vi "Set Alternating BD Colours.vi"(8 "error in (no error)":errorcluster, 11 "VI Path":path) -> (0 "error out":errorcluster)   [LabVIEW 2020]
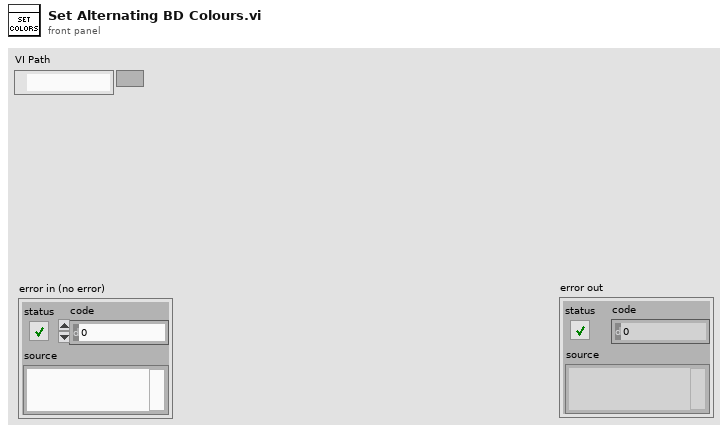
[diagram p1: front panel]
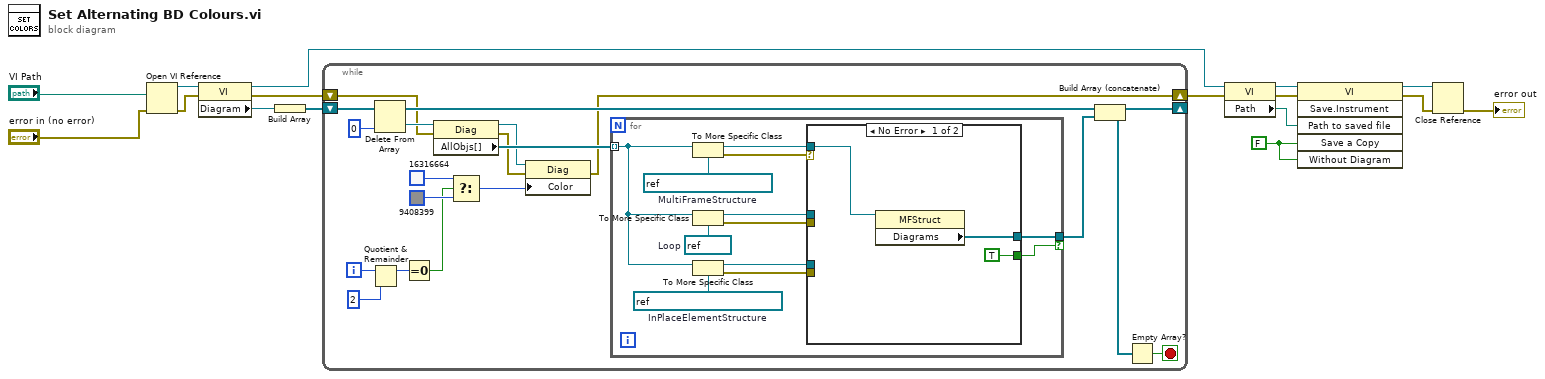
[diagram p0: block diagram]
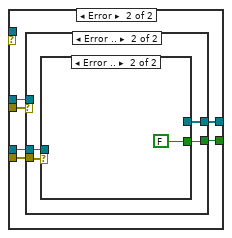
[diagram p2: hidden frame]
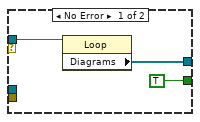
[diagram p3: hidden frame]
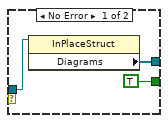
[diagram p4: hidden frame]
diagram:
  w5 = FALSE
  n1 = Open VI Reference(vi path="VI Path", error in (no error)="error in (no error)") -> (vi reference=w15:refnum<vi>, error out=w12:errorcluster)  [unwired: 4 in]
  n2 = property class="VI"(reference=w15, error in=w12) -> (reference out=w9:refnum<vi>, error out=w11:errorcluster, "Diagram"=w14:refnum<vi>)
  n3 = Build Array(w14) -> (w13:refnum<vi>[])
  n4 = while {
    shift-right: [w28] -> _
    shift-left: w13 -> [w35]
    shift-right: [w17] -> w10
    shift-left: w11 -> [w19]
    i -> [w27]
    stop <- w29 stop-if-true
    n5 = Quotient & Remainder(x=w27, y=2) -> (x-y*floor(x/y)=w23:i32)  [unwired: 1 out]
    n6 = Delete From Array(array=w35, index=0) -> (deleted portion=w33:refnum<vi>, array with subset deleted=w31:refnum<vi>[])  [unwired: 1 in]
    n7 = Equal To 0?(x=w23) -> (x = 0?=w22:bool)
    n8 = property class="Diag"(reference=w33, error in=w19) -> (reference out=w21:refnum<vi>, error out=w18:errorcluster, "AllObjs[]"=w32:refnum<vi>[])
    n9 = Select(t=u32 16316664, s=w22, f=u32 9408399) -> (s? t:f=w20:u32)
    n10 = property class="Diag"(reference=w21, error in=w18, "Color"=w20) -> (error out=w17:errorcluster)  [unwired: 1 out]
    n11 = for {
      tunnel: w32 -> [w44] mode=indexing
      tunnel: [w37] -> w30 if=w36
      w45 = refnum<vi> refnum  # InPlaceElementStructure
      w46 = refnum<vi> refnum  # Loop
      w47 = refnum<vi> refnum  # MultiFrameStructure
      n12 = To More Specific Class(target class=w47, reference=w44) -> (specific class reference=w42:refnum<vi>, error out=w43:errorcluster)  [unwired: 1 in]
      n13 = To More Specific Class(target class=w46, reference=w44) -> (specific class reference=w40:refnum<vi>, error out=w41:errorcluster)  [unwired: 1 in]
      n14 = To More Specific Class(target class=w45, reference=w44) -> (specific class reference=w38:refnum<vi>, error out=w39:errorcluster)  [unwired: 1 in]
      n15 = case shown="No Error" w43 {
        tunnel: w42 -> [w50 _]
        tunnel: w41 -> [_ w56]
        tunnel: w40 -> [_ w55]
        tunnel: w39 -> [_ w52]
        tunnel: w38 -> [_ w51]
        tunnel: [w49 w54] -> w37
        tunnel: [TRUE w53] -> w36
        frame No Error {
          n16 = property class="MFStruct"(reference=w50) -> ("Diagrams"=w49:refnum<vi>[])  [unwired: 1 in, 2 out]
        }
        frame Error {
          n17 = case shown="Error .." w56 {
            tunnel: w55 -> [w59 _]
            tunnel: [w58 w61] -> w54
            tunnel: [TRUE w60] -> w53
            tunnel: w52 -> [_ w63]
            tunnel: w51 -> [_ w62]
            frame No Error {
              n18 = property class="Loop"(reference=w59) -> ("Diagrams"=w58:refnum<vi>[])  [unwired: 1 in, 2 out]
            }
            frame Error {
              n19 = case shown="Error .." w63 {
                tunnel: w62 -> [w66 _]
                tunnel: [w65 _] -> w61
                tunnel: [TRUE FALSE] -> w60
                frame No Error {
                  n20 = property class="InPlaceStruct"(reference=w66) -> ("Diagrams"=w65:refnum<vi>[])  [unwired: 1 in, 2 out]
                }
                frame Error {
                }
              }
            }
          }
        }
      }
    }
    n21 = Build Array (concatenate)(w31, w30) -> (w28:refnum<vi>[])
    n22 = Empty Array?(array=w28) -> (empty?=w29:bool)
  }
  n23 = property class="VI"(reference=w9, error in=w10) -> (reference out=w7:refnum<vi>, error out=w8:errorcluster, "Path"=w6:path)
  n24 = invoke class="VI" method="Save.Instrument"(reference=w7, error in=w8, "Path to saved file"=w6, "Save a Copy"=w5, "Without Diagram"=w5) -> (reference out=w4:refnum<vi>, error out=w3:errorcluster)  [unwired: 1 in, 4 out]
  n25 = Close Reference(reference=w4, error in (no error)=w3) -> (error out=→"error out":errorcluster)
